vi "测试.vi"() -> ()   [LabVIEW 2014, in "DetecElecXControl.xctl"]
uses:
  DetecElecXControl.xctl
panel:
  in  "DetecElecXControl":T1(xcontrol)
  in  "不显示":bool
  in  "显示":bool
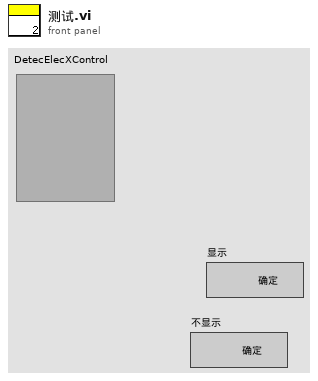
[diagram p1: front panel]
types:
  T1 = cluster{"Data":bool, "ElecName":string, "mapX":string, "mapY":string, "VV":string}
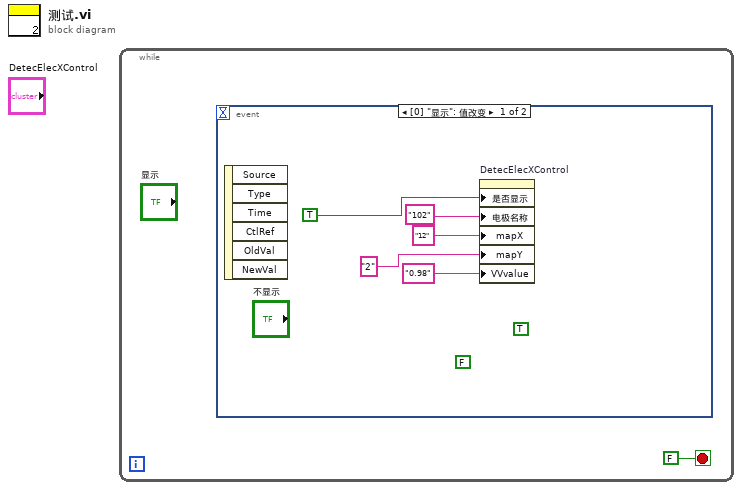
[diagram p0: block diagram]
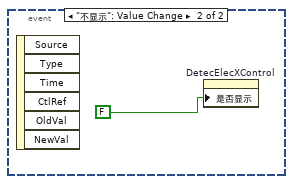
[diagram p2: hidden frame]
diagram:
  (unwired) TRUE ("显示")
  n1 = while {
    stop <- FALSE stop-if-true
    n2 = event shown="[0] \"显示\": 值改变" {
      selector: _ -> [_ _]
      dyn-events: _ -> [_ _]
      timeout: _ -> [_ _]
      event "显示": Value Change {
        (unwired) FALSE ("显示")
        n3 = event-data() -> ()  [unwired: 1 in, 6 out]
        n4 = property on="DetecElecXControl" class="DetecElecXControl (严格)"("是否显示"=TRUE, "电极名称"="102", "mapX"="12", "mapY"="2", "VVvalue"="0.98") -> ()  [unwired: 2 in, 2 out]
      }
      event "不显示": Value Change {
        n5 = event-data() -> ()  [unwired: 1 in, 6 out]
        n6 = property on="DetecElecXControl" class="DetecElecXControl (严格)"("是否显示"=FALSE) -> ()  [unwired: 2 in, 2 out]
      }
    }
  }
